vi "SetdBBoost.vi"(8 "错误输入（无错误）":errorcluster, 10 "使能":i32) -> (0 "错误输出":errorcluster)   [LabVIEW 2014]
uses:
  X86Dll/ZXUTConfigMgr.dll
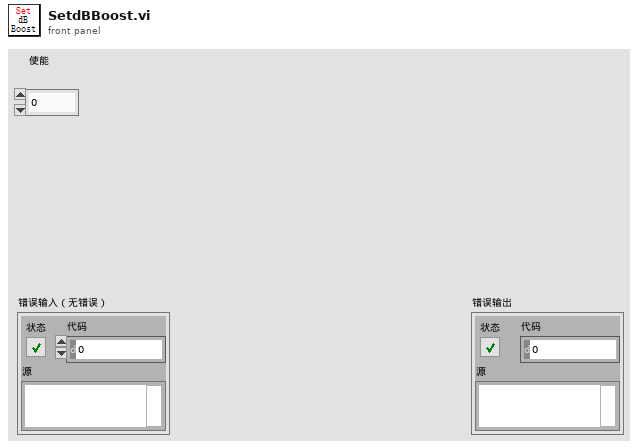
[diagram p1: front panel]
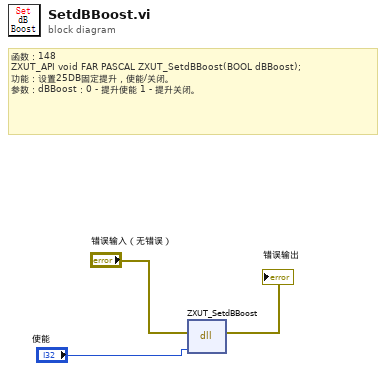
[diagram p0: block diagram]
diagram:
  # "函数：148\nZXUT_API void\tFAR PASCAL ZXUT_SetdBBoost(BOOL dBBoost);\n功能：设置25DB固定提升，使能/关闭。\n参数：dBBoost：0 - 提升使能 1 - 提升关闭。"
  n1 = dll-call lib="D:/Software/Utrasonic on-line monitoring/X86Dll/ZXUTConfigMgr.dll" fn="ZXUT_SetdBBoost"(error in="错误输入（无错误）", "dBBoost"="使能") -> (error out=→"错误输出":errorcluster)  [unwired: 4 in, 1 out]
